vi "logEventTask.vi"(8 "error in (no error)":errorcluster, 9 "pathOfSubEventSummaryState":path, 10 "pathLvLib":path, 11 "pathMonitor":path) -> (0 "error out":errorcluster)   [LabVIEW 2018]
doc: "Task of logging the event of LabVIEW. The event message is received by the CPP."
uses:
  SalProcess/SalProcess.lvclass
  LibReader/LibReader.lvclass
  SalProcess/SalProcess.lvclass/SalProcess.ctl
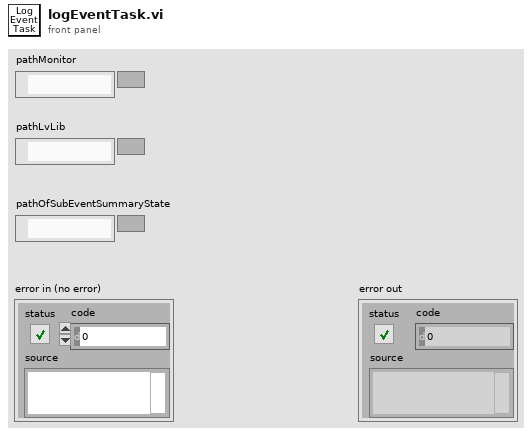
[diagram p1: front panel]
types:
  T1 = typedef "summaryState.ctl" = enum16{"", "DisabledState", "EnabledState", "FaultState", "OfflineState", "StandbyState"}
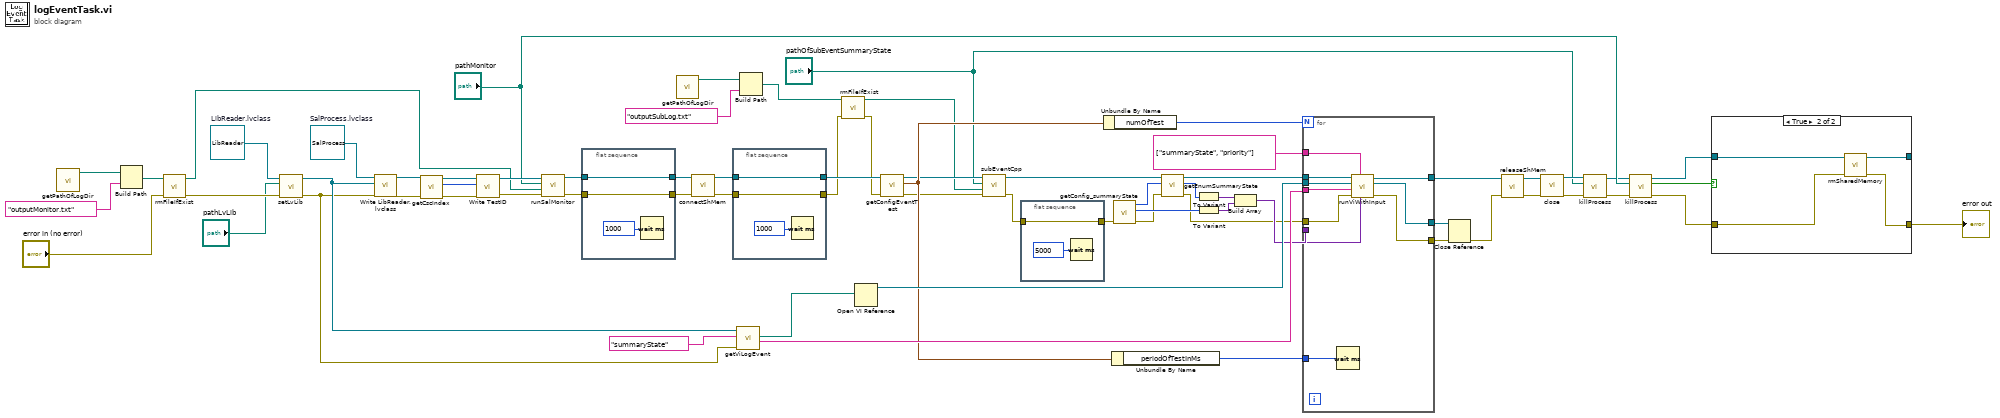
[diagram p0: block diagram]
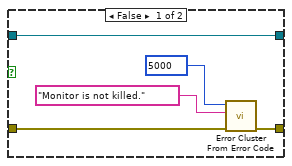
[diagram p2: hidden frame]
diagram:
  w56 = refnum<class "LibReader.lvclass"> refnum  # LibReader.lvclass
  w55 = refnum<class "SalProcess.lvclass"> refnum  # SalProcess.lvclass
  n1 = call "getPathOfLogDir.vi"() -> ("logDirPath"=w69:path)  [unwired: 11 in]
  n2 = Build Path(base path=w69, name or relative path="outputMonitor.txt") -> (appended path=w67:path)
  n3 = call "rmFileIfExist.vi"("error in (no error)"="error in (no error)", "path"=w67) -> ("error out"=w54:errorcluster, "pathDup"=w63:path)  [unwired: 8 in]
  n4 = call "setLvLib.vi"("error in (no error)"=w54, "pathLvLib"="pathLvLib", "LibReader in"=w56) -> ("error out"=w38:errorcluster, "LibReader out"=w40:refnum<class "LibReader.lvclass">)  [unwired: 7 in]
  n5 = call "Write LibReader.lvclass.vi"("error in (no error)"=w38, "LibReader.lvclass"=w40, "SalProcess in"=w55) -> ("error out"=w41:errorcluster, "SalProcess out"=w45:refnum<class "SalProcess.lvclass">)  [unwired: 7 in]
  n6 = call "getCscIndex.vi"("error in (no error)"=w41, "SalProcess in"=w45) -> ("error out"=w42:errorcluster, "cscIdx"=w43:i32, "SalProcess out"=w44:refnum<class "SalProcess.lvclass">)  [unwired: 7 in]
  n7 = call "Write TestID.vi"("error in (no error)"=w42, "TestID"=w43, "SalProcess in"=w44) -> ("error out"=w64:errorcluster, "SalProcess out"=w65:refnum<class "SalProcess.lvclass">)  [unwired: 7 in]
  n8 = call "runSalMonitor.vi"("error in (no error)"=w64, "pathOfOutput"=w63, "pathOfSalMonitor"="pathMonitor", "SalProcess in"=w65) -> ("error out"=w62:errorcluster, "SalProcess out"=w61:refnum<class "SalProcess.lvclass">)  [unwired: 6 in]
  n9 = flat-sequence {
    tunnel: w62 -> [w72]
    tunnel: w61 -> [w70]
    tunnel: [w72] -> w50
    tunnel: [w70] -> w51
    frame #0 {
      n10 = Wait (ms)(milliseconds to wait=u32 1000) -> ()  [unwired: 1 out]
    }
  }
  n11 = call "getPathOfLogDir.vi"() -> ("logDirPath"=w22:path)  [unwired: 11 in]
  n12 = call "connectShMem.vi"("error in (no error)"=w50, "SalProcess in"=w51) -> ("error out"=w49:errorcluster, "SalProcess out"=w48:refnum<class "SalProcess.lvclass">)  [unwired: 7 in, 1 out]
  n13 = flat-sequence {
    tunnel: w49 -> [w74]
    tunnel: w48 -> [w75]
    tunnel: [w75] -> w32
    tunnel: [w74] -> w18
    frame #0 {
      n14 = Wait (ms)(milliseconds to wait=u32 1000) -> ()  [unwired: 1 out]
    }
  }
  n15 = call "getViLogEvent.vi"("error in (no error)"=w38, "name"="summaryState", "LibReader in"=w40) -> ("clusterNameInput"=w33:string, "pathViLogEvent"=w37:path)  [unwired: 5 in, 2 out]
  n16 = Build Path(base path=w22, name or relative path="outputSubLog.txt") -> (appended path=w20:path)
  n17 = call "rmFileIfExist.vi"("error in (no error)"=w18, "path"=w20) -> ("error out"=w17:errorcluster, "pathDup"=w19:path)  [unwired: 8 in]
  n18 = Open VI Reference(vi path=w37) -> (vi reference=w36:refnum<vi>)  [unwired: 5 in, 1 out]
  n19 = call "getConfigEventTest.vi"("error in (no error)"=w17, "SalProcess in"=w32) -> ("error out"=w28:errorcluster, "configEventTest"=w31:cluster{"numOfTest":i32, "periodOfTestInMs":u32}, "SalProcess out"=w29:refnum<class "SalProcess.lvclass">)  [unwired: 7 in]
  n20 = call "subEventCpp.vi"("error in (no error)"=w28, "pathOfOutput"=w19, "pathOfSubEvent"="pathOfSubEventSummaryState", "SalProcess in"=w29) -> ("error out"=w7:errorcluster, "SalProcess out"=w6:refnum<class "SalProcess.lvclass">)  [unwired: 5 in, 1 out]
  n21 = flat-sequence {
    tunnel: [w77] -> w8
    tunnel: w7 -> [w77]
    frame #0 {
      n22 = Wait (ms)(milliseconds to wait=u32 5000) -> ()  [unwired: 1 out]
    }
  }
  n23 = Unbundle By Name(w31) -> ("numOfTest"=w14:i32)
  n24 = Unbundle By Name(w31) -> ("periodOfTestInMs"=w30:u32)
  n25 = call "getConfig_summaryState.vi"("error in (no error)"=w8) -> ("error out"=w2:errorcluster, "priority"=w13:i32, "summaryState"=w4:i32)  [unwired: 8 in]
  n26 = call "getEnumSummaryState.vi"("error in (no error)"=w2, "valSummaryState"=w4, "SalProcess in"=w6) -> ("error out"=w1:errorcluster, "enumSummaryState"=w3:T1, "SalProcess out"=w5:refnum<class "SalProcess.lvclass">)  [unwired: 6 in]
  n27 = To Variant(anything=w3) -> (Variant=w12:variant)
  n28 = To Variant(anything=w13) -> (Variant=w11:variant)
  n29 = Build Array(w12, w11) -> (w9:variant[])
  n30 = for {
    N: w14 -> [_]
    tunnel: w5 -> [w86]
    tunnel: [w80] -> w16
    tunnel: w36 -> [w84]
    tunnel: [w79] -> w35
    tunnel: [w81] -> w34
    tunnel: w33 -> [w83]
    tunnel: w30 -> [w87]
    tunnel: string[] ["summaryState", "priority"] -> [w85]
    tunnel: w9 -> [w82]
    tunnel: w1 -> [w78]
    n31 = Wait (ms)(milliseconds to wait=w87) -> ()  [unwired: 1 out]
    n32 = call "runViWithInput.vi"("valueElement"=w82, "nameElement"=w85, "error in (no error)"=w78, "clusterNameInput"=w83, "referenceIn"=w84, "SalProcess in"=w86) -> ("error out"=w81:errorcluster, "referenceOut"=w79:refnum<vi>, "SalProcess out"=w80:refnum<class "SalProcess.lvclass">)  [unwired: 3 in]
  }
  n33 = Close Reference(reference=w35, error in (no error)=w34) -> (error out=w15:errorcluster)
  n34 = call "releaseShMem.vi"("error in (no error)"=w15, "SalProcess in"=w16) -> ("error out"=w46:errorcluster, "SalProcess out"=w47:refnum<class "SalProcess.lvclass">)  [unwired: 7 in, 1 out]
  n35 = call "close.vi"("error in (no error)"=w46, "SalProcess in"=w47) -> ("error out"=w24:errorcluster, "SalProcess out"=w27:refnum<class "SalProcess.lvclass">)  [unwired: 8 in]
  n36 = call "killProcess.vi"("error in (no error)"=w24, "pathOfProcess"="pathOfSubEventSummaryState", "SalProcess in"=w27) -> ("error out"=w25:errorcluster, "SalProcess out"=w26:refnum<class "SalProcess.lvclass">)  [unwired: 6 in, 1 out]
  n37 = call "killProcess.vi"("error in (no error)"=w25, "pathOfProcess"="pathMonitor", "SalProcess in"=w26) -> ("error out"=w58:errorcluster, "isRemoved"=w60:bool, "SalProcess out"=w59:refnum<class "SalProcess.lvclass">)  [unwired: 6 in]
  n38 = case shown="True" w60 {
    tunnel: w59 -> [w92 w93]
    tunnel: w58 -> [w90 w94]
    tunnel: [w91 w96] -> w57
    tunnel: [w92 w95] -> _
    frame False {
      n39 = call <vilib>:"Error Cluster From Error Code.vi"("error in (no error)"=w90, "error message (\"\")"="Monitor is not killed." ("error message (\"\")"), "error code (0)"=5000) -> ("error out"=w91:errorcluster)  [unwired: 6 in]
    }
    frame True {
      n40 = call "rmSharedMemory.vi"("error in (no error)"=w94, "SalProcess in"=w93) -> ("error out"=w96:errorcluster, "SalProcess out"=w95:refnum<class "SalProcess.lvclass">)  [unwired: 7 in, 1 out]
    }
  }
  "error out" <- w57
